vi "Get Object Type.vi"(8 "error in":errorcluster, 11 "Object Entry in":refnum<class "Object Entry.lvclass">) -> (0 "error out":errorcluster, 2 "Object Type":T1={"Object Type"=0, "Null"=TRUE} {"Object Type" items=["NULL"=0, "DOMAIN"=2, "DEFTYPE"=5, "DEFSTRUCT"=6, "VAR"=7, "ARRAY"=8, "RECORD"=9]}, 3 "Object Entry out":refnum<class "Object Entry.lvclass">)   [LabVIEW 2019, in "Electronic Datasheet.lvlib" / "Object Entry.lvclass"]
uses:
  Object Entry.lvclass
  Object Entry.lvclass/Object Entry.ctl
  Object Type.ctl
  Electronic Datasheet.lvlib
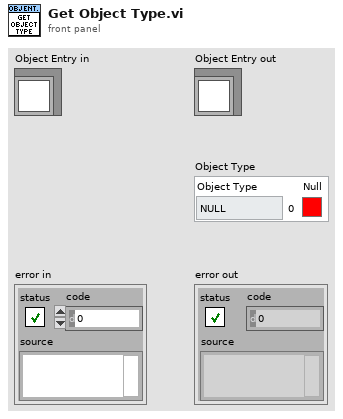
[diagram p1: front panel]
types:
  T1 = typedef "Electronic Datasheet.lvlib/Object Type.ctl" = cluster{"Object Type":u8, "Null":bool}
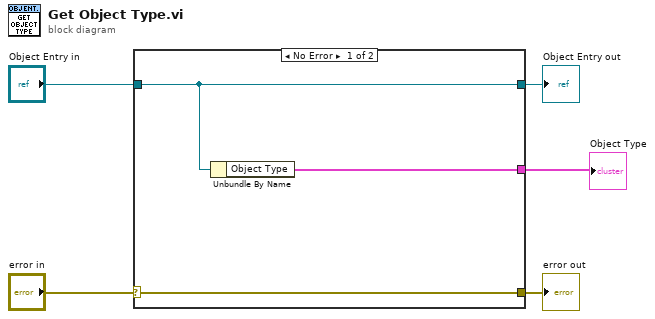
[diagram p0: block diagram]
diagram:
  n1 = case shown="No Error" "error in" {
    selector: "error in" -> [w8 w9]
    tunnel: [w8 w9] -> w4
    tunnel: [w7 w10] -> w2
    tunnel: "Object Entry in" -> [w7 w10]
    tunnel: [w6 _] -> w1
    frame No Error {
      n2 = Unbundle By Name(w7) -> ("Object Type"=w6:T1)
    }
    frame Error {
    }
  }
  "error out" <- w4
  "Object Entry out" <- w2
  "Object Type" <- w1
